vi "PH_StatusHandler.pack PSDB Data.vi"(0 "VI in":refnum<vi>, 2 "Replacements":cluster{"Status":T1, "String":string}[](array[cluster]) {"Status" items=["no info", "off/false/out", "on/true/in", "Failure", "Alarm", "Status 1", "Status 2", "Status 3"]}, 5 "error in (no error)":errorcluster) -> (14 "VI out":refnum<vi>, 16 "PSDB String Data Array":T2[](array[typedef]), 19 "error out":errorcluster)   [LabVIEW 2014, in "PH_StatusHandler.lvlib"]
doc: "This VI packs data for the PHELIX shot data base. Replacements may be used if certain Stati require another string."
uses:
  PH_StatusHandler.lvlib
  PH_PSDBWriter/PH_PSDBWriter.String dataset.ctl
  PH_StatusHandler.Status.ctl
  PH_PSDBWriter/PH_PSDBWriter.lvlib
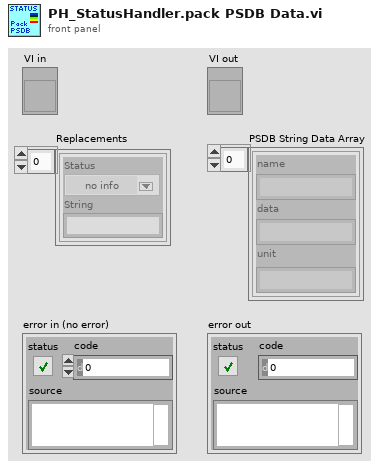
[diagram p1: front panel]
types:
  T1 = typedef "PH_StatusHandler.lvlib/PH_StatusHandler.Status.ctl" = i16
  T2 = typedef "PH_PSDBWriter.lvlib/PH_PSDBWriter.String dataset.ctl" = cluster{"name":string, "data":string, "unit":string}
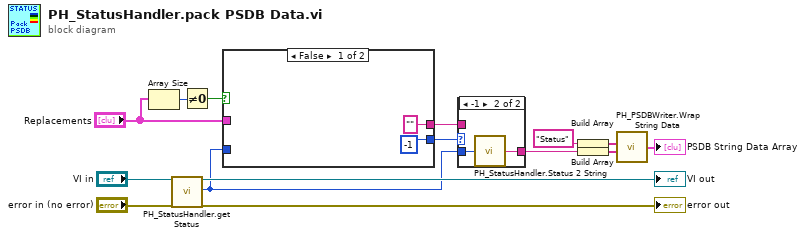
[diagram p0: block diagram]
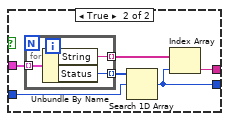
[diagram p2: hidden frame]
diagram:
  n1 = Array Size(array="Replacements") -> (size(s)=w3:i32)
  n2 = call "PH_StatusHandler.get Status.vi"("VI in"="VI in", "error in"="error in (no error)") -> ("VI out"=→"VI out":refnum<vi>, "Status"=w6:T1, "error out"=→"error out":errorcluster)  [unwired: 15 in]
  n3 = Not Equal To 0?(x=w3) -> (x != 0?=w4:bool)
  n4 = case shown="False" w4 {
    tunnel: "Replacements" -> [_ w23]
    tunnel: w6 -> [_ w21]
    tunnel: [-1 ("index of element") w19] -> w5
    tunnel: ["" ("String") w18] -> w1
    frame False {
    }
    frame True {
      n5 = for {
        tunnel: w23 -> [w26] mode=indexing
        tunnel: [w25] -> w22 mode=indexing
        tunnel: [w24] -> w20 mode=indexing
        n6 = Unbundle By Name(w26) -> ("String"=w24:string, "Status"=w25:T1)
      }
      n7 = Search 1D Array(1D array=w22, element=w21) -> (index of element=w19:i32)  [unwired: 1 in]
      n8 = Index Array(array=w20, index=w19) -> (element=w18:string)
    }
  }
  n9 = case shown="-1" w5 {
    tunnel: [w27 w29] -> w15
    tunnel: w6 -> [_ w28]
    tunnel: w1 -> [w27 _]
    frame Default {
    }
    frame -1 {
      n10 = call "PH_StatusHandler.Status 2 String.vi"("Status"=w28) -> ("Status as string"=w29:string)
    }
  }
  n11 = Build Array("Status" ("name")) -> (w12:string[])
  n12 = Build Array(w15) -> (w14:string[])
  n13 = call "PH_PSDBWriter.Wrap String Data.vi"("Data Array"=w14, "Name Array"=w12) -> ("PSDB String Data Array"=→"PSDB String Data Array":T2[])  [unwired: 2 in]
